vi "Configure Preferences File1.vi"(8 "error in (no error)":errorcluster, 9 "File Name ()":string, 10 "Operation (0: Load Preferences)":i32(ring) items=["Load Preferences", " Store Preferences"], 11 "VISA resource name":refnum<visa-resource-name>) -> (0 "error out":errorcluster, 3 "VISA resource name out":refnum<visa-resource-name>)   [LabVIEW 2015, in "Agilent 3446X Series1.lvlib"]
doc: "Configures the preferences file."
uses:
  Agilent 3446X Series1.lvlib
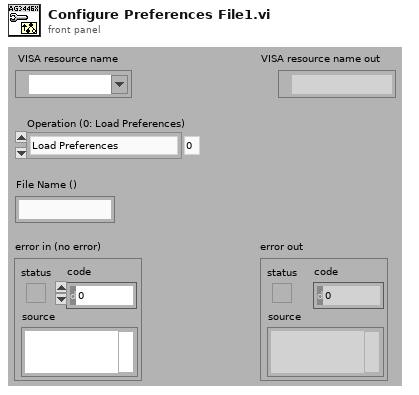
[diagram p1: front panel]
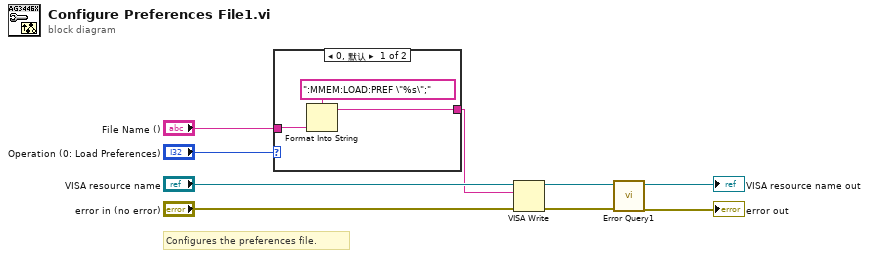
[diagram p0: block diagram]
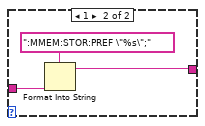
[diagram p2: hidden frame]
diagram:
  # "Configures the preferences file."
  n1 = case shown="0, 默认" "Operation (0: Load Preferences)" {
    tunnel: "File Name ()" -> [w11 w13]
    tunnel: [w10 w14] -> w1
    frame 0, Default {
      n2 = Format Into String(format string=":MMEM:LOAD:PREF \"%s\";", w11) -> (resulting string=w10:string)  [unwired: 2 in, 1 out]
    }
    frame 1 {
      n3 = Format Into String(format string=":MMEM:STOR:PREF \"%s\";", w13) -> (resulting string=w14:string)  [unwired: 2 in, 1 out]
    }
  }
  n4 = VISA Write(VISA resource name="VISA resource name", write buffer=w1, error in (no error)="error in (no error)") -> (VISA resource name out=w7:refnum<visa-resource-name>, error out=w6:errorcluster)  [unwired: 1 out]
  n5 = call "Error Query1.vi"("error in (no error)"=w6, "VISA resource name"=w7) -> ("error out"=→"error out":errorcluster, "VISA resource name out"=→"VISA resource name out":refnum<visa-resource-name>)  [unwired: 8 out]
